vi "data buffer.vi"(4 "Error In":errorcluster) -> (0 "Error Out":errorcluster, 3 "DVR":refnum<data-value>)   [LabVIEW 2015, in "Ramp Signal Data Buffer.lvlib"]
uses:
  Ramp Signal Data Buffer.lvlib
  buffer data typedef.ctl
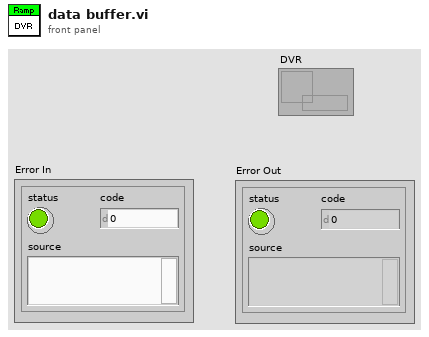
[diagram p1: front panel]
types:
  T1 = typedef "Ramp Signal Data Buffer.lvlib/buffer data typedef.ctl" = cluster{"Ramp Data":dbl[], "Counter":i32}
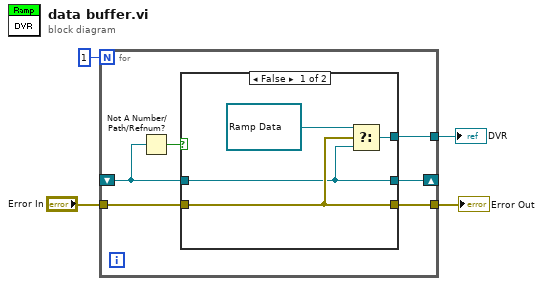
[diagram p0: block diagram]
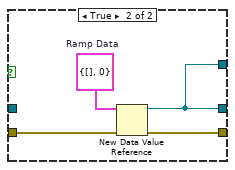
[diagram p2: hidden frame]
diagram:
  n1 = for {
    N: 1 -> [_]
    tunnel: "Error In" -> [w10]
    tunnel: [w9] -> w3
    shift-right: [w8] -> _
    shift-left: _ -> [w6]
    tunnel: [w5] -> w1
    n2 = Not A Number/Path/Refnum?(number/path/refnum=w6) -> (NaN/Path/Refnum?=w7:bool)
    n3 = case shown="False" w7 {
      tunnel: w10 -> [w14 w17]
      tunnel: [w14 w16] -> w9
      tunnel: [w13 w15] -> w8
      tunnel: w6 -> [w13 _]
      tunnel: [w12 w15] -> w5
      frame False {
        n4 = Select(t=refnum<data-value> refnum, s=w14, f=w13) -> (s? t:f=w12:refnum<data-value>)
      }
      frame True {
        w18 = T1 {"Ramp Data"=[], "Counter"=0}  # Ramp Data
        n5 = New Data Value Reference(data value=w18, error in=w17) -> (data value reference=w15:refnum<data-value>, error out=w16:errorcluster)
      }
    }
  }
  "Error Out" <- w3
  "DVR" <- w1
